vi "GetAutotoolRegions.vi"(0 "XRef":T17, 1 "State In":T7) -> (14 "Regions":T2, 15 "Fatal Error Out":T1)   [LabVIEW 2020, in "Parallel Diagram Block.xnode"]
uses:
  Parallel Diagram Block.xnode
  <vilib>/XNodeSupport/XNodeXNodeRef.ctl
  State.ctl
  Parallel Block/Type Descriptor.ctl
  Parallel Block/Direction.ctl
  Parallel Block/Value Type.ctl
  Parallel Block/Terminal Mode.ctl
  Parallel Block/Terminal Type.ctl
  <vilib>/picture/picture.llb/imagedata.ctl
  <vilib>/XNodeSupport/XNodeAutotoolRegions.ctl
  <vilib>/XNodeSupport/XNodeAutotoolRegion.ctl
  <vilib>/XNodeSupport/XNodeRect32.ctl
  <vilib>/XNodeSupport/XNodeInt.ctl
  <vilib>/XNodeSupport/XNodeTools.ctl
  <vilib>/XNodeSupport/XNodeErrorCluster.ctl
  <vilib>/XNodeSupport/NI_XNodeSupport.lvlib
  Parallel Block/Parallel Block.lvlib
  Parallel Block/Type Mode.ctl
  Parallel Block/Value Mode.ctl
  Parallel Block/Manager Node.ctl
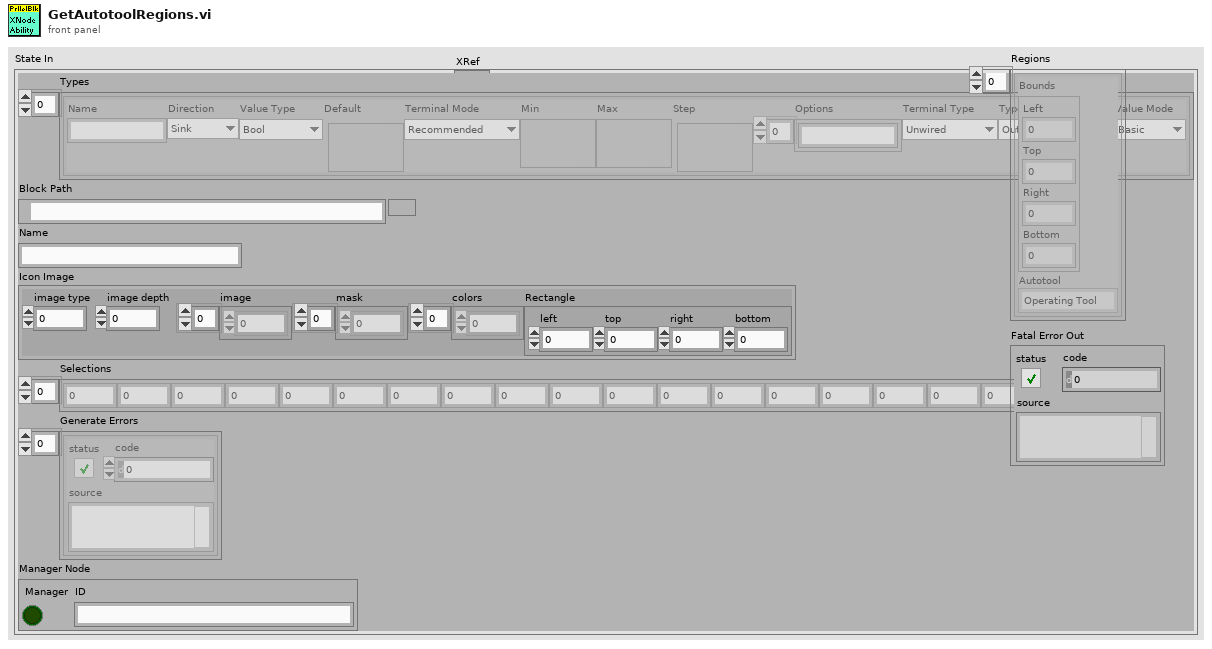
[diagram p1: front panel]
types:
  T1 = typedef "NI_XNodeSupport.lvlib/XNodeErrorCluster.ctl" = errorcluster
  T2 = typedef "NI_XNodeSupport.lvlib/XNodeAutotoolRegions.ctl" = T3[]
  T3 = typedef "NI_XNodeSupport.lvlib/XNodeAutotoolRegion.ctl" = cluster{"Bounds":T4, "Autotool":T6}
  T4 = typedef "NI_XNodeSupport.lvlib/XNodeRect32.ctl" = cluster{"Left":T5, "Top":T5, "Right":T5, "Bottom":T5}
  T5 = typedef "NI_XNodeSupport.lvlib/XNodeInt.ctl" = i32
  T6 = typedef "NI_XNodeSupport.lvlib/XNodeTools.ctl" = enum32{"Operating Tool", "Placement Tool", "Labelling Tool", "Wiring Tool", "Scroll Tool", "Breakpoint Tool", "Probe Tool", "Auto Tool"}
  T7 = typedef "Parallel Diagram Block.xnode/State.ctl" = cluster{"Types":T8[], "Block Path":path, "Name":string, "Icon Image":T15, "Selections":i32[], "Generate Errors":errorcluster[], "Manager Node":T16}
  T8 = typedef "Parallel Block.lvlib/Type Descriptor.ctl" = cluster{"Name":string, "Direction":T9, "Value Type":T10, "Default":variant, "Terminal Mode":T11, "Min":variant, "Max":variant, "Step":variant, "Options":string[], "Terminal Type":T12, "Type Mode":T13, "Value Mode":T14}
  T9 = typedef "Parallel Block.lvlib/Direction.ctl" = enum16{"Sink", "Source"}
  T10 = typedef "Parallel Block.lvlib/Value Type.ctl" = enum16{"Unknown", "Bool", "U8", "U16", "U32", "U64", "I8", "I16", "I32", "I64", "SGL", "DBL", "CSG", "CDB", "CDBWfm", "String", "DBLWfm"}
  T11 = typedef "Parallel Block.lvlib/Terminal Mode.ctl" = enum16{"Recommended", "Required", "None"}
  T12 = typedef "Parallel Block.lvlib/Terminal Type.ctl" = enum16{"Unwired", "BadType", "Connection", "Value", "Control Ref", "BadRefType"}
  T13 = typedef "Parallel Block.lvlib/Type Mode.ctl" = enum16{"Output", "Single - Strict", "Single - Coerced", "Stream"}
  T14 = typedef "Parallel Block.lvlib/Value Mode.ctl" = enum16{"Basic", "Range", "Select"}
  T15 = typedef "imagedata.ctl" = cluster{"image type":i32, "image depth":i32, "image":u8[], "mask":u8[], "colors":u32[], "Rectangle":cluster{"left":i16, "top":i16, "right":i16, "bottom":i16}}
  T16 = typedef "Parallel Block.lvlib/Manager Node.ctl" = cluster{"Manager":bool, "ID":string}
  T17 = typedef "NI_XNodeSupport.lvlib/XNodeXNodeRef.ctl" = refnum<vi>
  T18 = cluster{"left":i16, "top":i16, "right":i16, "bottom":i16}
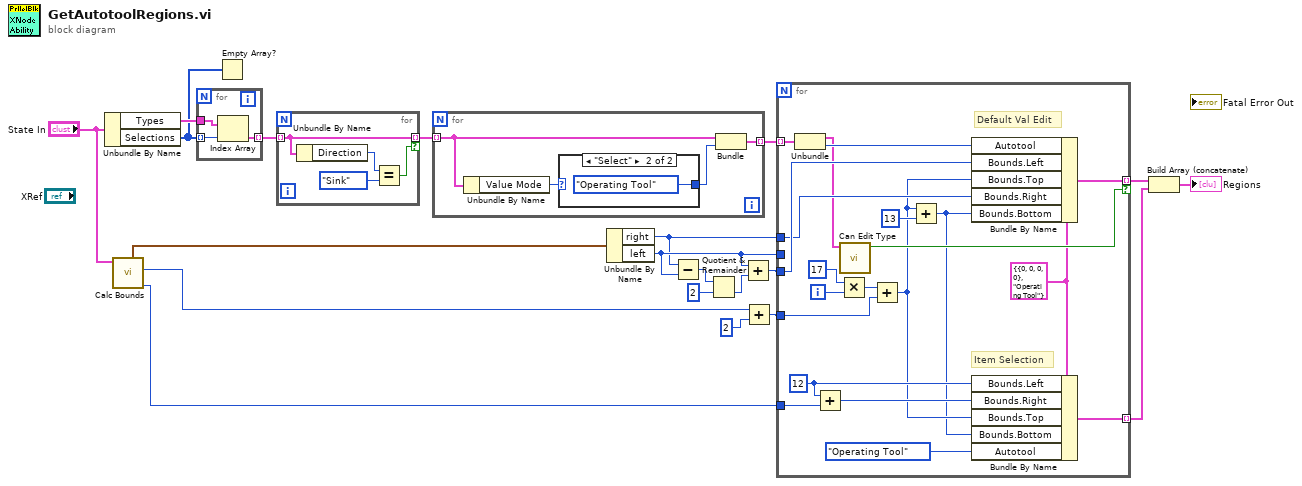
[diagram p0: block diagram]
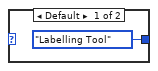
[diagram p2: hidden frame]
diagram:
  n1 = Unbundle By Name("State In") -> ("Types"=w8:T8[], "Selections"=w6:i32[])
  n2 = call "Calc Bounds.vi"("State"="State In") -> ("Name Width"=w1:i16, "Header"=w5:i32, "Bounds Without Terminals"=w18:T18)  [unwired: 4 in, 4 out]
  n3 = for {
    tunnel: w8 -> [w23]
    tunnel: w6 -> [w22] mode=indexing
    tunnel: [w21] -> w7 mode=indexing
    n4 = Index Array(array=w23, index=w22) -> (element=w21:T8)
  }
  n5 = Empty Array?(array=w6) -> ()  [unwired: 1 out]
  n6 = for {
    tunnel: w7 -> [w25] mode=indexing
    tunnel: [w25] -> w9 mode=indexing if=w24
    n7 = Unbundle By Name(w25) -> ("Direction"=w26:T9)
    n8 = Equal?(x=w26, y=Direction."Sink" ("Direction")) -> (x = y?=w24:bool)
  }
  n9 = for {
    tunnel: w9 -> [w28] mode=indexing
    tunnel: [w29] -> w19 mode=indexing
    n10 = Unbundle By Name(w28) -> ("Value Mode"=w31:T14)
    n11 = case shown="\"Select\"" w31 {
      tunnel: [XNodeTools."Labelling Tool" ("Autotool") XNodeTools."Operating Tool" ("Autotool")] -> w30
      frame Default {
      }
      frame "Select" {
      }
    }
    n12 = Bundle("Type Descriptor"=w28, "Autotool"=w30) -> (w29:cluster{"Type Descriptor":T8, "Autotool":T6})  [unwired: 1 in]
  }
  n13 = Unbundle By Name(w18) -> ("right"=w12:i16, "left"=w13:i16)
  n14 = Subtract(x=w12, y=w13) -> (x-y=w17:i16)
  n15 = Quotient & Remainder(x=w17, y=i16 2) -> (floor(x/y)=w15:i16)  [unwired: 1 out]
  n16 = Add(x=w13, y=w15) -> (x+y=w14:i16)
  n17 = Add(x=w5, y=2) -> (x+y=w11:i32)
  n18 = for {
    tunnel: w19 -> [w53] mode=indexing
    tunnel: w14 -> [w51]
    tunnel: w13 -> [_]
    tunnel: w12 -> [w50]
    tunnel: [w52] -> w4 mode=indexing if=w42
    tunnel: w11 -> [w46]
    tunnel: [w41] -> w2 mode=indexing
    tunnel: w1 -> [w39]
    i -> [w49]
    w38 = T5 12 ("Bounds.Left")
    w40 = T3 {"Bounds"={"Left"=0, "Top"=0, "Right"=0, "Bottom"=0}, "Autotool"=enum."Operating Tool"} ("Autotool Region")
    # "Default Val Edit"
    # "Item Selection"
    n19 = Unbundle(w53) -> ("Type Descriptor"=w43:T8, "Autotool"=w44:T6)
    n20 = Add(x=w38, y=w39) -> (x+y=w37:T5)
    n21 = Multiply(x=17, y=w49) -> (x*y=w47:i32)
    n22 = call "Can Edit Type.vi"("Type Descriptor"=w43) -> ("Can Edit?"=w42:bool)  [unwired: 10 in]
    n23 = Add(x=w47, y=w46) -> (x+y=w36:i32)
    n24 = Add(x=w36, y=13) -> (x+y=w35:i32)
    n25 = Bundle By Name(cluster=w40, "Autotool"=w44, "Bounds.Left"=w51, "Bounds.Top"=w36, "Bounds.Right"=w50, "Bounds.Bottom"=w35) -> (w52:T3)
    n26 = Bundle By Name(cluster=w40, "Bounds.Left"=w38, "Bounds.Right"=w37, "Bounds.Top"=w36, "Bounds.Bottom"=w35, "Autotool"=XNodeTools."Operating Tool") -> (w41:T3)
  }
  n27 = Build Array (concatenate)(w4, w2) -> (→"Regions":T3[])
